vi "Read XNET.vi"(8 "error in":errorcluster, 11 "PCAN in":refnum<class "PCAN.lvclass">) -> (0 "error out":errorcluster, 3 "PCAN out":refnum<class "PCAN.lvclass">)   [LabVIEW 2023, in "PCAN.lvclass"]
uses:
  PCAN.lvclass
  PCAN.lvclass/PCAN.ctl
  <vilib>/xnet/xnet.llb/XNET Frame Type CAN.ctl
  <vilib>/xnet/xnet.llb/XNET Convert (Frame CAN to Signal).vi
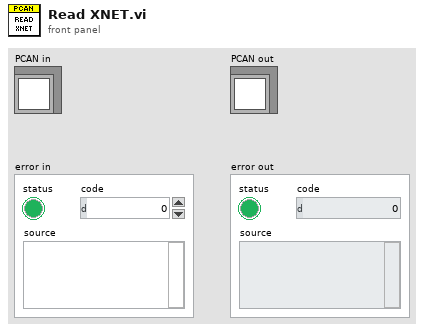
[diagram p1: front panel]
types:
  T1 = typedef "TPCANHandle.ctl" = enum16{"PCAN_NONEBUS  0x000", "PCAN_ISABUS1  0x21", "PCAN_ISABUS2  0x22", "PCAN_ISABUS3  0x23", "PCAN_ISABUS4  0x24", "PCAN_ISABUS5  0x25", "PCAN_ISABUS6  0x26", "PCAN_ISABUS7  0x27", "PCAN_ISABUS8  0x28", "PCAN_DNGBUS1  0x31", "PCAN_PCIBUS1  0x41", "PCAN_PCIBUS1  0x42", "PCAN_PCIBUS1  0x43", "PCAN_PCIBUS1  0x44", "PCAN_PCIBUS1  0x45", "PCAN_PCIBUS1  0x46", "PCAN_PCIBUS1  0x47", "PCAN_PCIBUS1  0x48", "PCAN_PCIBUS1  0x409", "PCAN_PCIBUS1  0x40A", "PCAN_PCIBUS1  0x40B", "PCAN_PCIBUS1  0x40C", "PCAN_PCIBUS1  0x40D", "PCAN_PCIBUS1  0x40E", "PCAN_PCIBUS1  0x40F", "PCAN_PCIBUS1  0x410", "PCAN_USBBUS1  0x51", "PCAN_USBBUS2  0x52", "PCAN_USBBUS3  0x53", "PCAN_USBBUS4  0x54", "PCAN_USBBUS5  0x55", "PCAN_USBBUS6  0x56", "PCAN_USBBUS7  0x57", "PCAN_USBBUS8  0x58", "PCAN_USBBUS9  0x509", "PCAN_USBBUS10  0x50A", "PCAN_USBBUS11  0x50B", "PCAN_USBBUS12  0x50C", "PCAN_USBBUS13  0x50D", "PCAN_USBBUS14  0x50E", "PCAN_USBBUS15  0x50F", "PCAN_USBBUS16  0x510", "PCAN_PCCBUS1  0x61", "PCAN_PCCBUS2  0x62", "PCAN_LANBUS1  0x801", "PCAN_LANBUS2  0x802", "PCAN_LANBUS3  0x803", "PCAN_LANBUS4  0x804", "PCAN_LANBUS5  0x805", "PCAN_LANBUS6  0x806", "PCAN_LANBUS7  0x807", "PCAN_LANBUS8  0x808", "PCAN_LANBUS9  0x809", "PCAN_LANBUS10  0x80A", "PCAN_LANBUS11  0x80B", "PCAN_LANBUS12  0x80C", "PCAN_LANBUS13  0x80D", "PCAN_LANBUS14  0x80E", "PCAN_LANBUS15  0x80F", "PCAN_LANBUS16  0x810"}
  T2 = typedef "TPCANTimestamp.ctl" = cluster{"millis overflow":u16, "millis ":u32, "micros":u16}
  T3 = typedef "CAN MSG Cluster.ctl" = cluster{"ID":u32, "MSG type":u8, "DLC":u8, "DATA":u8[]}
  T4 = typedef "XNET Frame Type CAN.ctl" = u8
  T5 = cluster{"timestamp":timestamp, "payload":u8[], "identifier":u32, "type":T4, "extended?":bool, "echo?":bool}
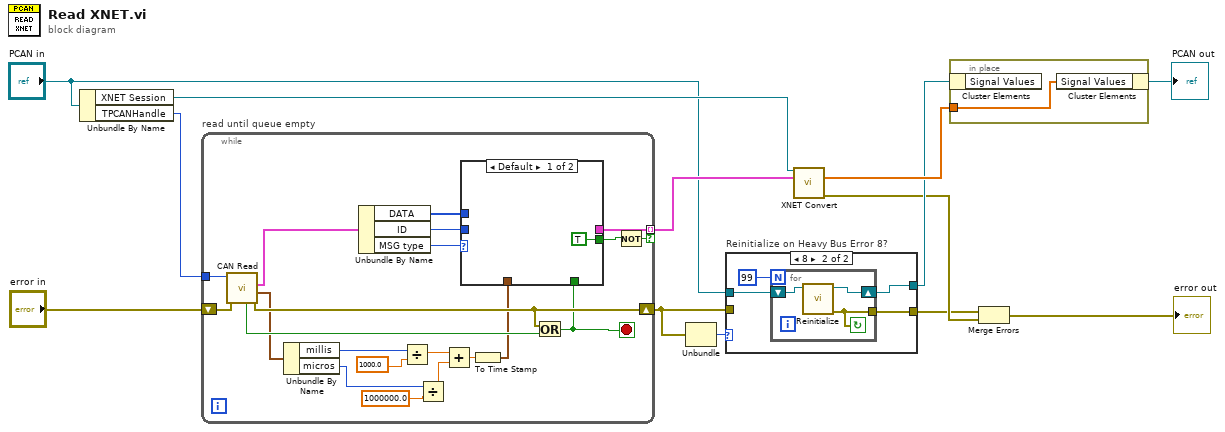
[diagram p0: block diagram]
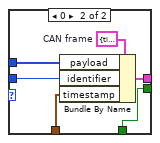
[diagram p3: hidden frame]
diagram:
  n1 = Unbundle By Name("PCAN in") -> ("XNET Session"=w11:refnum<k21>, "TPCANHandle"=w10:T1)
  n2 = while "read until queue empty" {
    tunnel: w10 -> [w34]
    shift-right: [w31] -> w4
    shift-left: "error in" -> [w33]
    tunnel: [w17] -> w12 mode=indexing if=w30
    stop <- w14 stop-if-true
    n3 = call <instrlib>:"CAN Read.vi"("error in (no error)"=w33, "TPCANHandle"=w34) -> ("error out"=w31:errorcluster, "TPCANTimestamp out"=w26:T2, "CAN_Message out"=w29:T3, "rcv queue empty"=w32:bool)  [unwired: 5 in, 1 out]
    n4 = Unbundle By Name(w26) -> ("millis"=w25:u32, "micros"=w23:u16)
    n5 = Unbundle By Name(w29) -> ("DATA"=w28:u8[], "ID"=w27:u32, "MSG type"=w16:u8)
    n6 = Divide(x=w25, y=1000.0) -> (x/y=w19:dbl)
    n7 = Divide(x=w23, y=1000000.0) -> (x/y=w20:dbl)
    n8 = Add(x=w19, y=w20) -> (x+y=w21:dbl)
    n9 = To Time Stamp(1:w21) -> (0:w18:timestamp)
    n10 = Or(x=w31, y=w32) -> (x .or. y?=w14:bool)
    n11 = case shown="Default" w16 {
      tunnel: w28 -> [_ w40]
      tunnel: w27 -> [_ w39]
      tunnel: w18 -> [_ w38]
      tunnel: [_ w37] -> w17
      tunnel: [TRUE w36] -> w15
      tunnel: w14 -> [_ w36]
      frame Default {
      }
      frame 0 {
        w41 = T5 {"timestamp"=timestamp(0 s since 1904-01-01), "payload"=[], "identifier"=0, "type"=0, "extended?"=FALSE, "echo?"=FALSE}  # CAN frame
        n12 = Bundle By Name(cluster=w41, "payload"=w40, "identifier"=w39, "timestamp"=w38) -> (w37:T5)
      }
    }
    n13 = Not(x=w15) -> (.not. x?=w30:bool)
  }
  n14 = Unbundle(w4) -> ("code"=w7:i32)  [unwired: 2 out]
  n15 = case "Reinitialize on Heavy Bus Error 8?" shown="8" w7 {
    tunnel: [w43 w47] -> w2
    tunnel: w4 -> [w43 _]
    tunnel: "PCAN in" -> [w42 w46]
    tunnel: [w42 w45] -> w5
    frame Default {
    }
    frame 8 {
      n16 = for {
        N: 99 -> [_]
        tunnel: [w48] -> w47
        shift-right: [w49] -> w45
        shift-left: w46 -> [w50]
        stop <- w48 continue-if-true
        n17 = call "Reinitialize.vi"("PCAN in"=w50) -> ("error out"=w48:errorcluster, "PCAN out"=w49:refnum<class "PCAN.lvclass">)  [unwired: 9 in]
      }
    }
  }
  n18 = call-poly <vilib>:"XNET Convert.vi"("session in"=w11, "frame data"=w12) -> ("signal data"=w9:dbl[], "error out"=w3:errorcluster)  [unwired: 11 in, 1 out]
  n19 = in-place {
    in-place-border: w9 -> [w51]
    n20 = in-place-cluster #1(w5) -> ()  [unwired: 1 out]
    n21 = in-place-cluster #1("Signal Values"=w51) -> (→"PCAN out":refnum<class "PCAN.lvclass">)
  }
  n22 = Merge Errors(w2, w3) -> (→"error out":errorcluster)
